vi "ModifyNumberforFormat.vi"(11 "String to modify":string) -> (0 "Modified string":string, 3 "Format":string)   [LabVIEW 2011, in "Agilent 546XX Series.lvlib"]
uses:
  Agilent 546XX Series.lvlib
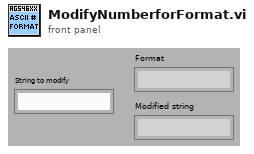
[diagram p1: front panel]
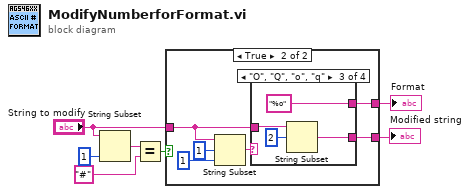
[diagram p0: block diagram]
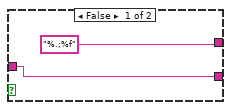
[diagram p2: hidden frame]
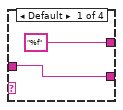
[diagram p3: hidden frame]
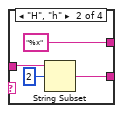
[diagram p4: hidden frame]
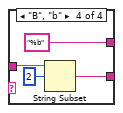
[diagram p5: hidden frame]
diagram:
  n1 = String Subset(string="String to modify", length (rest)=1 ("length (rest)")) -> (substring=w6:string)  [unwired: 1 in]
  n2 = Equal?(x=w6, y="#") -> (x = y?=w4:bool)
  n3 = case shown="True" w4 {
    tunnel: "String to modify" -> [w8 w10]
    tunnel: [w8 w12] -> w2
    tunnel: ["%.;%f" w11] -> w1
    frame False {
    }
    frame True {
      n4 = String Subset(string=w10, offset (0)=1, length (rest)=1 ("length (rest)")) -> (substring=w13:string)
      n5 = case shown="\"O\", \"Q\", \"o\", \"q\"" w13 {
        tunnel: [w16 w20 w24 w28] -> w12
        tunnel: ["%f" "%x" "%o" "%b"] -> w11
        tunnel: w10 -> [w16 w18 w22 w26]
        frame Default {
        }
        frame "H", "h" {
          n6 = String Subset(string=w18, offset (0)=2) -> (substring=w20:string)  [unwired: 1 in]
        }
        frame "O", "Q", "o", "q" {
          n7 = String Subset(string=w22, offset (0)=2) -> (substring=w24:string)  [unwired: 1 in]
        }
        frame "B", "b" {
          n8 = String Subset(string=w26, offset (0)=2) -> (substring=w28:string)  [unwired: 1 in]
        }
      }
    }
  }
  "Modified string" <- w2
  "Format" <- w1
